vi "Drive_Arcade.vi"(3 "Joystick_In":T1) -> (0 "Right_Motor_Out":dbl, 1 "Left_Motor_Out":dbl)   [LabVIEW 2016]
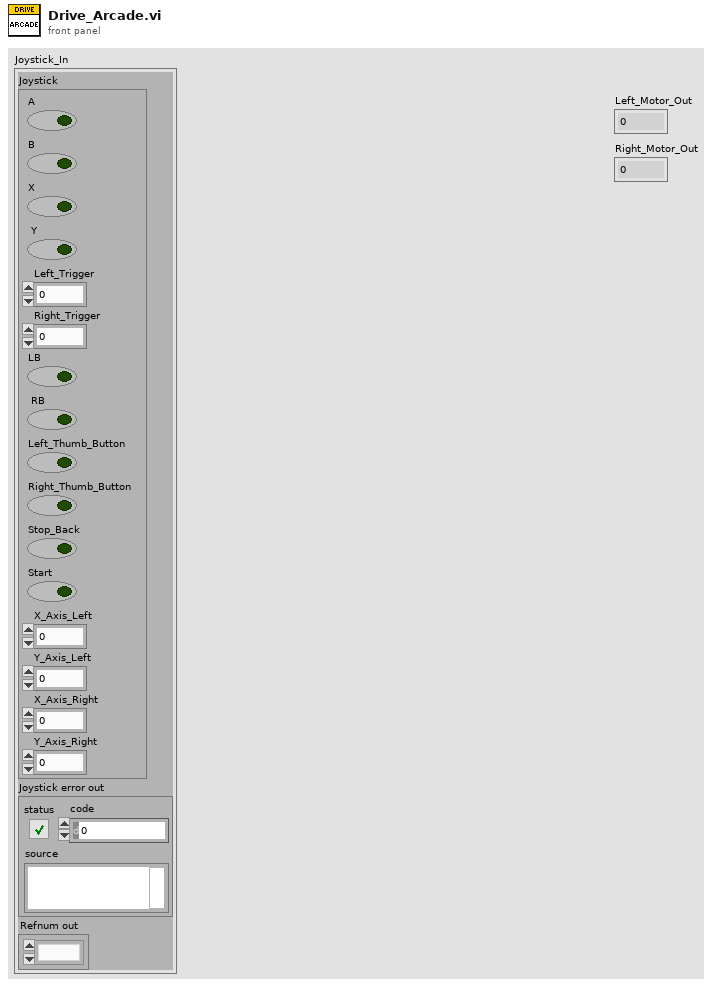
[diagram p1: front panel]
types:
  T1 = cluster{"Joystick":cluster{"A":bool, "B":bool, "X":bool, " Y":bool, "Left_Trigger":dbl, "Right_Trigger ":dbl, "LB":bool, " RB":bool, "Left_Thumb_Button":bool, "Right_Thumb_Button":bool, "Stop_Back":bool, "Start":bool, "X_Axis_Left":dbl, "Y_Axis_Left":dbl, "X_Axis_Right":dbl, "Y_Axis_Right":dbl}, "Joystick error out":errorcluster, "Refnum out":refnum<k1>}
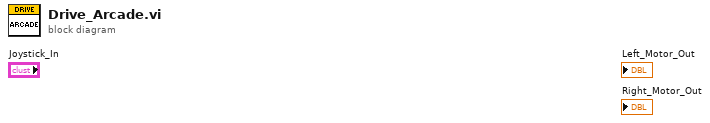
[diagram p0: block diagram]
diagram:
